vi "creditUpdate.vi"(8 "error in (no error)":errorcluster, 10 "Credit":dbl, 11 "UI Actor in":refnum<class "UI Actor.lvclass">) -> (0 "error out":errorcluster, 3 "UI Actor out":refnum<class "UI Actor.lvclass">)   [LabVIEW 2020, in "UI Actor.lvlib" / "UI Actor.lvclass"]
uses:
  UI Actor.lvclass
  UI Actor.lvclass/UI Actor.ctl
  MSG Messages/Update MSG Msg/Update MSG Msg.lvclass/Update MSG Msg.ctl
  <vilib>/ActorFramework/Message Enqueuer/Message Enqueuer.lvclass/Message Enqueuer.ctl
  <vilib>/ActorFramework/Message Enqueuer/Enqueue.vi
  MSG Messages/Update MSG Msg/Update MSG Msg.lvclass
  C:/Program Files (x86)/National Instruments/LabVIEW 2020/vi.lib/ActorFramework/Message/Message.lvclass
  <vilib>/ActorFramework/Message Priority Queue/Priority Enqueue.vi
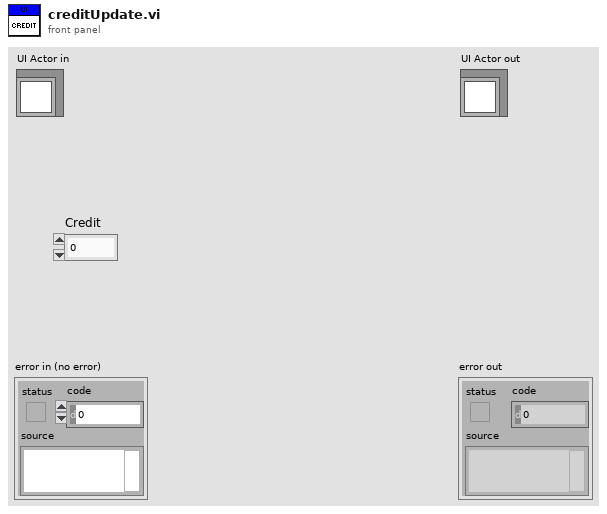
[diagram p1: front panel]
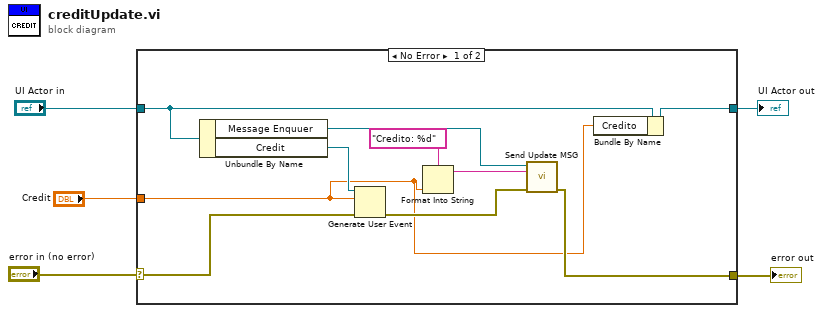
[diagram p0: block diagram]
diagram:
  n1 = case shown="No Error" "error in (no error)" {
    selector: "error in (no error)" -> [w13 w17]
    tunnel: [w10 w17] -> w4
    tunnel: [w7 w16] -> w2
    tunnel: "UI Actor in" -> [w15 w16]
    tunnel: "Credit" -> [w6 _]
    frame No Error {
      n2 = Unbundle By Name(w15) -> ("Message Enquuer"=w12:refnum<class "Message Enqueuer.lvclass">, "Credit"=w14:refnum<user-event>)
      n3 = Generate User Event(user event=w14, event data cluster=w6, error in=w13) -> (error out=w11:errorcluster)  [unwired: 1 in, 1 out]
      n4 = Format Into String(format string="Credito: %d", w6) -> (resulting string=w9:string)  [unwired: 2 in, 1 out]
      n5 = call "Send Update MSG.vi"("error in (no error)"=w11, "Update message"=w9, "Message Enqueuer"=w12) -> ("error out"=w10:errorcluster)  [unwired: 7 in, 1 out]
      n6 = Bundle By Name(cluster=w15, "Credito"=w6) -> (w7:refnum<class "UI Actor.lvclass">)
    }
    frame Error {
    }
  }
  "error out" <- w4
  "UI Actor out" <- w2
